vi "Destroy Events.vi"(8 "error in (no error)":errorcluster, 11 "uService Template in":refnum<class "Father of all uServices.lvclass">) -> (0 "error out":errorcluster, 3 "uService Template out":refnum<class "Father of all uServices.lvclass">)   [LabVIEW 2026, in "TALOS.lvlib" / "Father of all uServices.lvlib" / "Father of all uServices.lvclass"]
uses:
  Father of all uServices.lvclass
  <vilib>/event_ctls.llb/usereventprio.ctl
  Father of all uServices.lvclass/Father of all uServices.ctl
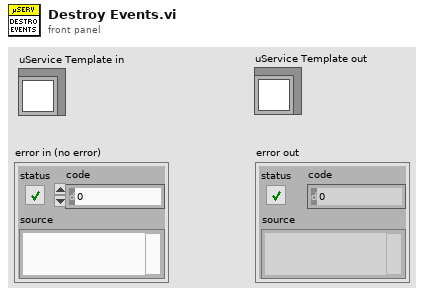
[diagram p1: front panel]
types:
  T1 = typedef "usereventprio.ctl" = enum32{"high priority", "normal priority"}
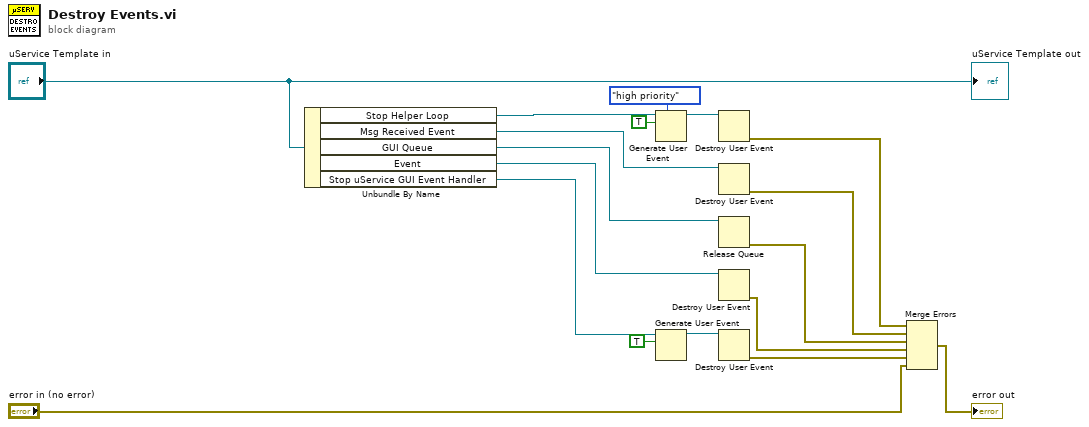
[diagram p0: block diagram]
diagram:
  n1 = Unbundle By Name("uService Template in") -> ("Stop Helper Loop"=w18:refnum<user-event>, "Msg Received Event"=w15:refnum<user-event>, "GUI Queue"=w11:refnum<queue>, "Event"=w9:refnum<user-event>, "Stop uService GUI Event Handler"=w5:refnum<user-event>)
  n2 = Generate User Event(priority (normal)=usereventprio."high priority", user event=w18, event data cluster=TRUE ("event data")) -> (user event out=w17:refnum<user-event>)  [unwired: 1 in, 1 out]
  n3 = Generate User Event(user event=w5, event data cluster=TRUE ("event data")) -> (user event out=w6:refnum<user-event>)  [unwired: 2 in, 1 out]
  n4 = Destroy User Event(user event=w17) -> (error out=w12:errorcluster)  [unwired: 1 in]
  n5 = Destroy User Event(user event=w15) -> (error out=w13:errorcluster)  [unwired: 1 in]
  n6 = Release Queue(queue=w11) -> (error out=w10:errorcluster)  [unwired: 2 in, 2 out]
  n7 = Destroy User Event(user event=w9) -> (error out=w8:errorcluster)  [unwired: 1 in]
  n8 = Destroy User Event(user event=w6) -> (error out=w4:errorcluster)  [unwired: 1 in]
  n9 = Merge Errors(w12, w13, w10, w8, w4, "error in (no error)") -> (→"error out":errorcluster)
  "uService Template out" <- "uService Template in"
